vi "RutaUDL.vi"() -> ()   [LabVIEW 2018]
panel:
  in  "Ruta UDL":path
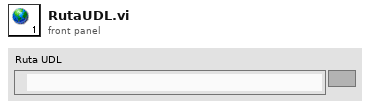
[diagram p1: front panel]
diagram:
